vi "Test 3.vi"() -> ()   [LabVIEW 2019]
uses:
  <vilib>/Powertrain Controls/Device Drivers/Engine Position Tracking/EPTx/RevA/RT/Controls/Settings - Pattern.ctl
  <vilib>/Powertrain Controls/Device Drivers/Engine Position Tracking/EPTx/RevA/RT/Controls/EPTxPattern.ctl
  <vilib>/Powertrain Controls/Device Drivers/Engine Position Tracking/EPTx/RevA/RT/Controls/Pattern.ctl
  <vilib>/Powertrain Controls/Device Drivers/Engine Position Tracking/EPTx/RevA/RT/Controls/EPTxSettings.ctl
  <vilib>/Powertrain Controls/Device Drivers/Engine Position Tracking/EPTx/RevA/RT/Controls/Settings - Tooth.ctl
  <vilib>/Powertrain Controls/Device Drivers/Engine Position Tracking/EPTx/RevA/RT/Controls/Direction Detection.ctl
  <vilib>/Powertrain Controls/Device Drivers/Engine Position Tracking/EPTx/RevA/RT/Controls/Settings - Token.ctl
  <vilib>/Powertrain Controls/Device Drivers/Engine Position Tracking/EPTx/RevA/RT/Controls/Aux Signal.ctl
  <vilib>/Powertrain Controls/Device Drivers/Engine Position Tracking/EPTx/RevA/RT/Controls/Aux Type.ctl
  <vilib>/Powertrain Controls/Device Drivers/Engine Position Tracking/EPTx/RevA/RT/Controls/Aux Threshold.ctl
  <vilib>/Powertrain Controls/Device Drivers/Engine Position Tracking/EPTx/RevA/RT/EPTx - RevA - RT.lvlib
panel:
  out "EPTxPatternSettings":T1
  in  "Pattern Path":path
  in  "Load":bool
  out "数组（最后n个元素置于前端）":T3[](array[typedef]) {"dAngle" format="%#_10g"}
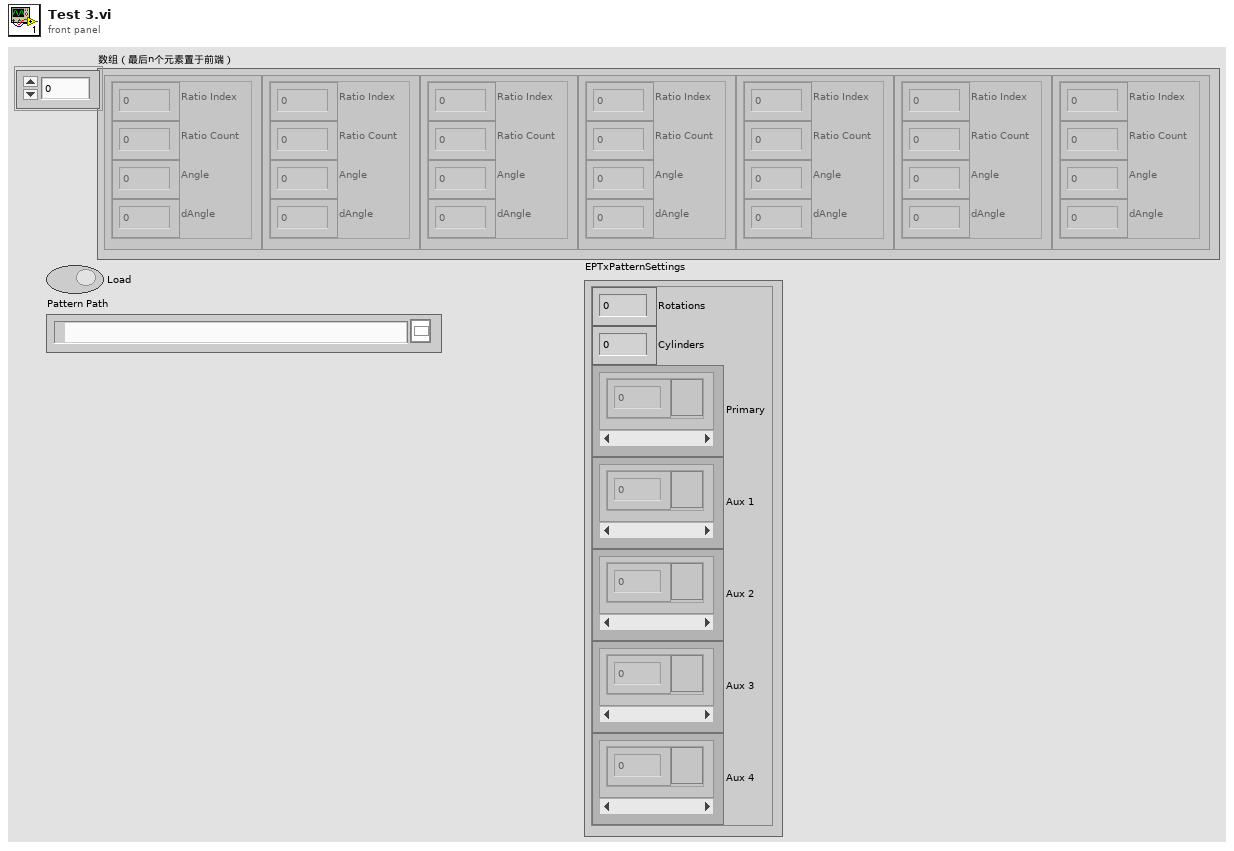
[diagram p1: front panel]
types:
  T1 = typedef "EPTx - RevA - RT.lvlib/EPTxPattern.ctl" = cluster{"Rotations":u8, "Cylinders":u8, "Primary":T2[], "Aux 1":T2[], "Aux 2":T2[], "Aux 3":T2[], "Aux 4":T2[]}
  T2 = typedef "EPTx - RevA - RT.lvlib/Pattern.ctl" = cluster{"Angle":sgl, "State":bool}
  T3 = typedef "EPTx - RevA - RT.lvlib/Settings - Pattern.ctl" = cluster{"Ratio Index":u8, "Ratio Count":u16, "Angle":sgl, "dAngle":sgl}
  T4 = typedef "EPTx - RevA - RT.lvlib/Aux Threshold.ctl" = cluster{"Aux 1":sgl, "Aux 2":sgl, "Aux 3":sgl, "Aux 4":sgl}
  T5 = typedef "EPTx - RevA - RT.lvlib/Settings - Tooth.ctl" = cluster{"Rising Edge":bool, "Falling Edge":bool, "Direction\nDetection":T6, "Level":bool, "Parameter":sgl}
  T6 = typedef "EPTx - RevA - RT.lvlib/Direction Detection.ctl" = enum16{"None", "Aux Signal", "Length"}
  T7 = typedef "EPTx - RevA - RT.lvlib/Settings - Token.ctl" = cluster{"Length":u16, "Start Index":u8, "Start Count":u16, "Aux 1":T8, "Aux 1 Type":T9, "Aux 1 Max":u16, "Aux 1 Min":u16, "Aux 2":T8, "Aux 2 Type":T9, "Aux 2 Max":u16, "Aux 2 Min":u16, "End Index":u8, "End Count":u16}
  T8 = typedef "EPTx - RevA - RT.lvlib/Aux Signal.ctl" = enum8{"---", "Aux 1", "Aux 2", "Aux 3", "Aux 4"}
  T9 = typedef "EPTx - RevA - RT.lvlib/Aux Type.ctl" = enum8{"Falling", "Rising", "Low", "High", "Ratio"}
  T10 = typedef "EPTx - RevA - RT.lvlib/EPTxSettings.ctl" = cluster{"Rotation":u8, "Ratios":sgl[], "Thresholds":sgl[], "Tooth":T5, "Pattern":T3[], "Token":T7[], "Aux Threshold Min":T4, "Aux Threshold Max":T4}
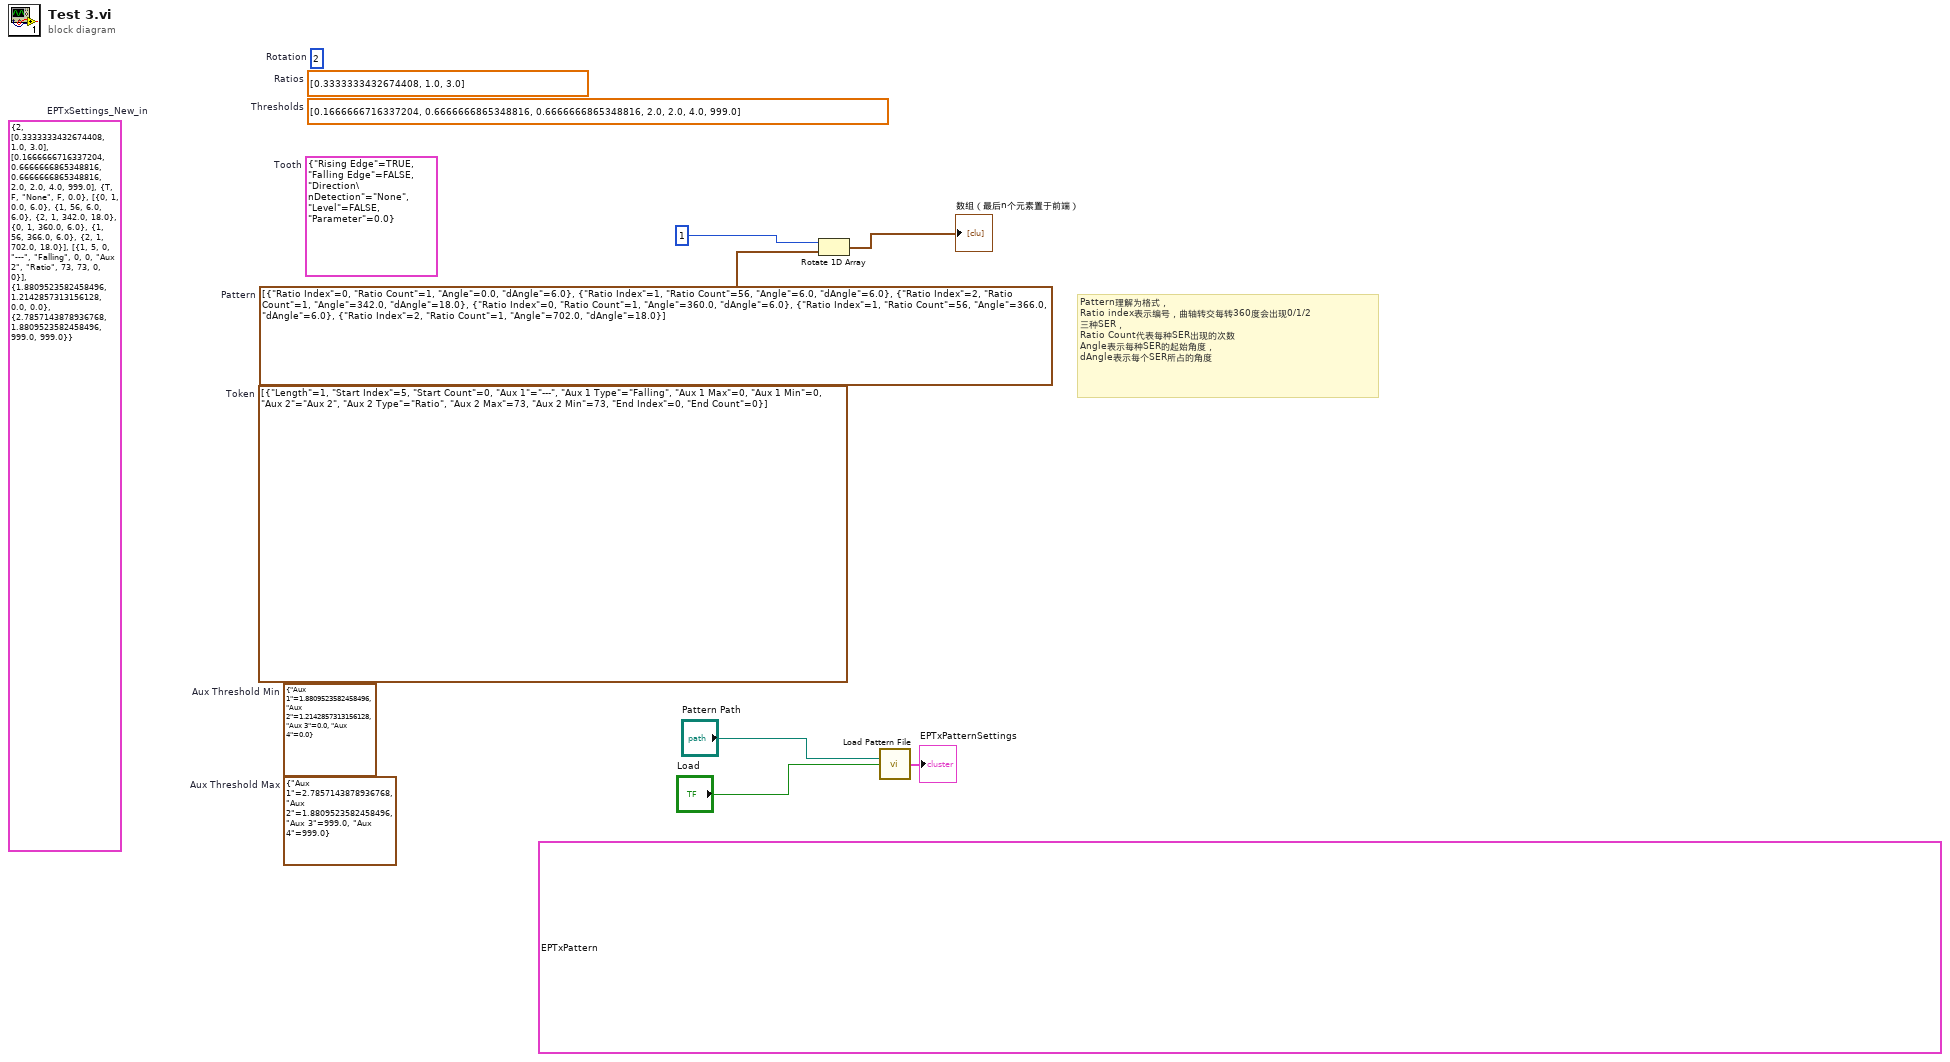
[diagram p0: block diagram]
diagram:
  (unwired) T1 data[8572B] ("EPTxPatternSettings")
  (unwired) T4 {"Aux 1"=2.7857144, "Aux 2"=1.8809524, "Aux 3"=999.0, "Aux 4"=999.0}  # Aux Threshold Max
  (unwired) T4 {"Aux 1"=1.8809524, "Aux 2"=1.2142857, "Aux 3"=0.0, "Aux 4"=0.0}  # Aux Threshold Min
  (unwired) u8 2  # Rotation
  (unwired) T5 {"Rising Edge"=TRUE, "Falling Edge"=FALSE, "Direction\nDetection"=enum."None", "Level"=FALSE, "Parameter"=0.0}  # Tooth
  (unwired) sgl[] [0.16666667, 0.6666667, 0.6666667, 2.0, 2.0, 4.0, 999.0]  # Thresholds
  (unwired) sgl[] [0.33333334, 1.0, 3.0]  # Ratios
  w6 = T3[] [{"Ratio Index"=0, "Ratio Count"=1, "Angle"=0.0, "dAngle"=6.0}, {"Ratio Index"=1, "Ratio Count"=56, "Angle"=6.0, "dAngle"=6.0}, {"Ratio Index"=2, "Ratio Count"=1, "Angle"=342.0, "dAngle"=18.0}, {"Ratio Index"=0, "Ratio Count"=1, "Angle"=360.0, "dAngle"=6.0}, {"Ratio Index"=1, "Ratio Count"=56, "Angle"=366.0, "dAngle"=6.0}, {"Ratio Index"=2, "Ratio Count"=1, "Angle"=702.0, "dAngle"=18.0}]  # Pattern
  (unwired) T7[] [{"Length"=1, "Start Index"=5, "Start Count"=0, "Aux 1"=enum."---", "Aux 1 Type"=enum."Falling", "Aux 1 Max"=0, "Aux 1 Min"=0, "Aux 2"=enum."Aux 2", "Aux 2 Type"=enum."Ratio", "Aux 2 Max"=73, "Aux 2 Min"=73, "End Index"=0, "End Count"=0}]  # Token
  (unwired) T10 {"Rotation"=2, "Ratios"=[0.33333334, 1.0, 3.0], "Thresholds"=[0.16666667, 0.6666667, 0.6666667, 2.0, 2.0, 4.0, 999.0], "Tooth"={"Rising Edge"=TRUE, "Falling Edge"=FALSE, "Direction\nDetection"=enum."None", "Level"=FALSE, "Parameter"=0.0}, "Pattern"=[{"Ratio Index"=0, "Ratio Count"=1, "Angle"=0.0, "dAngle"=6.0}, {"Ratio Index"=1, "Ratio Count"=56, "Angle"=6.0, "dAngle"=6.0}, {"Ratio Index"=2, "Ratio Count"=1, "Angle"=342.0, "dAngle"=18.0}, {"Ratio Index"=0, "Ratio Count"=1, "Angle"=360.0, "dAngle"=6.0}, {"Ratio Index"=1, "Ratio Count"=56, "Angle"=366.0, "dAngle"=6.0}, {"Ratio Index"=2, "Ratio Count"=1, "Angle"=702.0, "dAngle"=18.0}], "Token"=[{"Length"=1, "Start Index"=5, "Start Count"=0, "Aux 1"=enum."---", "Aux 1 Type"=enum."Falling", "Aux 1 Max"=0, "Aux 1 Min"=0, "Aux 2"=enum."Aux 2", "Aux 2 Type"=enum."Ratio", "Aux 2 Max"=73, "Aux 2 Min"=73, "End Index"=0, "End Count"=0}], "Aux Threshold Min"={"Aux 1"=1.8809524, "Aux 2"=1.2142857, "Aux 3"=0.0, "Aux 4"=0.0}, "Aux Threshold Max"={"Aux 1"=2.7857144, "Aux 2"=1.8809524, "Aux 3"=999.0, "Aux 4"=999.0}}  # EPTxSettings_New_in
  # "Pattern理解为格式，\nRatio index表示编号，曲轴转交每转360度会出现0/1/2\n三种SER，\nRatio Count代表每种SER出现的次数\nAngle表示每种SER的起始角度，\ndAngle表示每个SER所占的角度"
  n1 = Rotate 1D Array(1:w6, 2:1 ("n")) -> (0:→"数组（最后n个元素置于前端）":T3[])
  n2 = call <vilib>:"Load Pattern File.vi"("Pattern Path"="Pattern Path", "Load"="Load") -> ("EPTxPatternSettings"=→"EPTxPatternSettings":T1)  [unwired: 12 in, 1 out]
